vi "Array PLC Byte Stream to G Object.vi"(8 "error in (no error)":errorcluster, 9 "Array Type Descriptor":T1, 10 "Byte Stream":u8[](array[numeric]), 11 "TwinCAT ADS in":refnum<class "TwinCAT ADS.lvclass">) -> (0 "error out":errorcluster, 2 "Value":variant, 3 "TwinCAT ADS out":refnum<class "TwinCAT ADS.lvclass">)   [LabVIEW 2018, in "TwinCAT ADS.lvclass"]
uses:
  TwinCAT ADS.lvclass
  Controls/PLC Array Type Descriptor.ctl
  Controls/PLC Type.ctl
  Controls/PLC Sub-Item Type Descriptor.ctl
  Standard PLC Byte Stream to G Object.vi/9a8c356b-cf55-4838-9201-0532b80217b2.vi
  Standard PLC Byte Stream to G Object.vi/06482052-d1f9-4f29-aca9-908031c6a69f.vi
  Standard PLC Byte Stream to G Object.vi/b9242781-96b0-446e-9150-452b1084ed54.vi
  Standard PLC Byte Stream to G Object.vi/5fbe6976-0b86-40a2-b7b6-3748894f0071.vi
  Standard PLC Byte Stream to G Object.vi/c4de1741-fffd-4fed-ba25-d7b4acbf0555.vi
  Standard PLC Byte Stream to G Object.vi/20356124-05d2-4a04-a5d1-e69adc4c58c2.vi
  Standard PLC Byte Stream to G Object.vi/67ddb754-0fbe-43d9-9e61-34d6659124ef.vi
  Standard PLC Byte Stream to G Object.vi/e3d41cb3-d20e-45e9-8252-e41884a8f4d0.vi
  Standard PLC Byte Stream to G Object.vi/46ba2a54-cc07-4222-9a0e-bd972edfcef0.vi
  Standard PLC Byte Stream to G Object.vi/6b416cf7-30dc-48a3-9278-9d800f443678.vi
  Standard PLC Byte Stream to G Object.vi/5857d013-9824-4299-a2d7-53efdc0d26c5.vi
  Standard PLC Byte Stream to G Object.vi/006b0e7e-7e80-41f3-be4e-1f3da8479fae.vi
  Standard PLC Byte Stream to G Object.vi/28d9c90b-5f2a-4c58-95e2-5fc46303b0fd.vi
  Standard PLC Byte Stream to G Object.vi/99b7bc4a-962e-4818-aa5d-444f23f83b11.vi
  Standard PLC Byte Stream to G Object.vi/8b7c42c8-9170-4542-8f35-15cbeddc22cb.vi
  Standard PLC Byte Stream to G Object.vi/65a091fa-0bd2-4a35-ae2b-3fa5e90d1994.vi
  Standard PLC Byte Stream to G Object.vi/4b7d3a7d-7f1b-46f0-9357-48cb72148c56.vi
  Standard PLC Byte Stream to G Object.vi/b431183c-2ad5-4c6d-9bfa-a53b18913682.vi
  Standard PLC Byte Stream to G Object.vi/30c6c28a-53c3-4e33-80b1-b22f521e1f67.vi
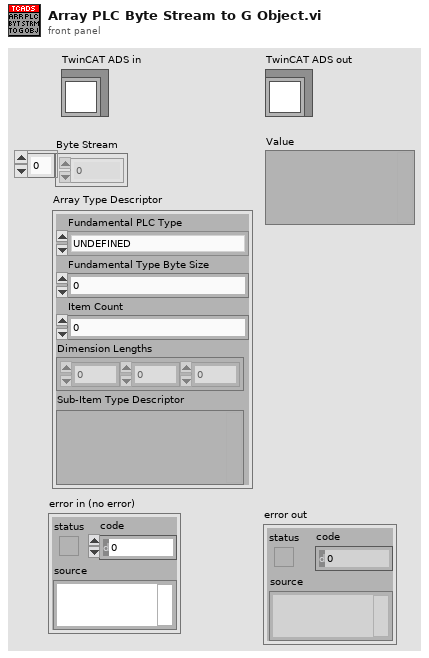
[diagram p1: front panel]
types:
  T1 = typedef "TwinCAT ADS.lvclass/PLC Array Type Descriptor.ctl" = cluster{"Fundamental PLC Type":T2, "Fundamental Type Byte Size":i32, "Item Count":i32, "Dimension Lengths":i32[], "Sub-Item Type Descriptor":variant}
  T2 = typedef "TwinCAT ADS.lvclass/PLC Type.ctl" = enum16{"UNDEFINED", "INT", "DINT", "REAL", "LREAL", "SINT", "BYTE", "UINT", "UDINT", "LINT", "ULINT", "STRING", "WSTRING", "BOOL", "TIME", "LTIME", "DATE", "DT", "TOD", "ARRAY", "JAGGED ARRAY", "STRUCT", "FUNCTION BLOCK", "POINTER", "USER DEFINED"}
  T3 = typedef "TwinCAT ADS.lvclass/PLC Sub-Item Type Descriptor.ctl" = cluster{"PLC Type":T2, "Offset":i32, "Byte Size":i32, "[Sub-Item/Array Type Descriptor]":variant[]}
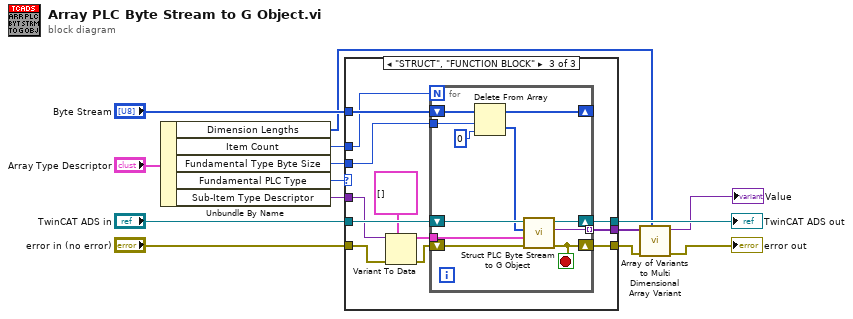
[diagram p0: block diagram]
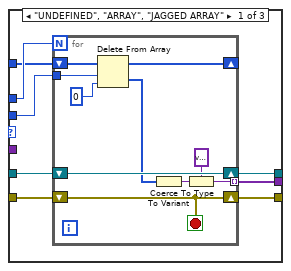
[diagram p2: hidden frame]
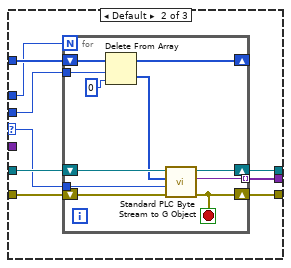
[diagram p3: hidden frame]
diagram:
  n1 = Unbundle By Name("Array Type Descriptor") -> ("Dimension Lengths"=w1:i32[], "Item Count"=w5:i32, "Fundamental Type Byte Size"=w3:i32, "Fundamental PLC Type"=w4:T2, "Sub-Item Type Descriptor"=w6:variant)
  n2 = case shown="\"STRUCT\", \"FUNCTION BLOCK\"" w4 {
    selector: w4 -> [_ w35 _]
    tunnel: "error in (no error)" -> [w22 w41 w57]
    tunnel: "TwinCAT ADS in" -> [w21 w40 w64]
    tunnel: "Byte Stream" -> [w17 w39 w61]
    tunnel: [w19 w38 w62] -> w8
    tunnel: [w15 w37 w60] -> w12
    tunnel: [w20 w36 w63] -> w10
    tunnel: w6 -> [_ _ w56]
    tunnel: w5 -> [w18 w34 w59]
    tunnel: w3 -> [w16 w33 w58]
    frame "UNDEFINED", "ARRAY", "JAGGED ARRAY" {
      n3 = for {
        N: w18 -> [_]
        shift-right: [w32] -> w20
        shift-left: w21 -> [w32]
        shift-right: [w26] -> _
        shift-left: w17 -> [w27]
        tunnel: w16 -> [w25]
        tunnel: [w23] -> w15 mode=indexing
        shift-right: [w31] -> w19
        shift-left: w22 -> [w31]
        stop <- w31 stop-if-true
        n4 = Delete From Array(array=w27, length=w25, index=0) -> (deleted portion=w24:u8[], array with subset deleted=w26:u8[])
        n5 = To Variant(anything=w24) -> (Variant=w29:variant)
        n6 = Coerce To Type(0:w29, 1:variant ("Value")) -> (2:w23:variant)
      }
    }
    frame Default {
      n7 = for {
        N: w34 -> [_]
        shift-right: [w50] -> w36
        shift-left: w40 -> [w51]
        shift-right: [w47] -> _
        shift-left: w39 -> [w48]
        tunnel: [w46] -> w37 mode=indexing
        tunnel: w35 -> [w44]
        tunnel: w33 -> [w43]
        shift-right: [w42] -> w38
        shift-left: w41 -> [w52]
        stop <- w42 stop-if-true
        n8 = Delete From Array(array=w48, length=w43, index=0) -> (deleted portion=w45:u8[], array with subset deleted=w47:u8[])
        n9 = call "Standard PLC Byte Stream to G Object.vi"("error in (no error)"=w52, "PLC Type"=w44, "Byte Stream"=w45, "TwinCAT ADS in"=w51) -> ("error out"=w42:errorcluster, "Value"=w46:variant, "TwinCAT ADS out"=w50:refnum<class "TwinCAT ADS.lvclass">)  [unwired: 5 in]
      }
    }
    frame "STRUCT", "FUNCTION BLOCK" {
      n10 = Variant To Data(error in=w57, type=T3[] [] ("[Sub-Item Type Information]"), Variant=w56) -> (data=w53:T3[], error out=w55:errorcluster)
      n11 = for {
        N: w59 -> [_]
        shift-right: [w74] -> w63
        shift-left: w64 -> [w75]
        shift-right: [w69] -> _
        shift-left: w61 -> [w71]
        tunnel: [w68] -> w60 mode=indexing
        tunnel: w58 -> [w67]
        tunnel: w53 -> [w66]
        shift-right: [w65] -> w62
        shift-left: w55 -> [w73]
        stop <- w65 stop-if-true
        n12 = Delete From Array(array=w71, length=w67, index=0) -> (deleted portion=w70:u8[], array with subset deleted=w69:u8[])
        n13 = call "Struct PLC Byte Stream to G Object.vi"("error in (no error)"=w73, "[Sub-Item Type Information]"=w66, "Byte Stream"=w70, "TwinCAT ADS in"=w75) -> ("error out"=w65:errorcluster, "Value"=w68:variant, "TwinCAT ADS out"=w74:refnum<class "TwinCAT ADS.lvclass">)  [unwired: 5 in]
      }
    }
  }
  "TwinCAT ADS out" <- w10
  n14 = call "Array of Variants to Multi Dimensional Array Variant.vi"("Dimension Lengths"=w1, "error in (no error)"=w8, "[Variant]"=w12) -> ("error out"=→"error out":errorcluster, "Array Variant"=→"Value":variant)  [unwired: 7 in]
